vi "zad2a.vi"() -> ()   [LabVIEW 2017]
uses:
  zad2Zmienna.vi
panel:
  out "Numeric":dbl
  in  "OK Button":bool
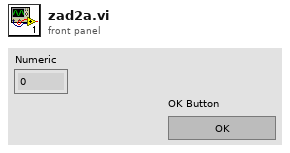
[diagram p1: front panel]
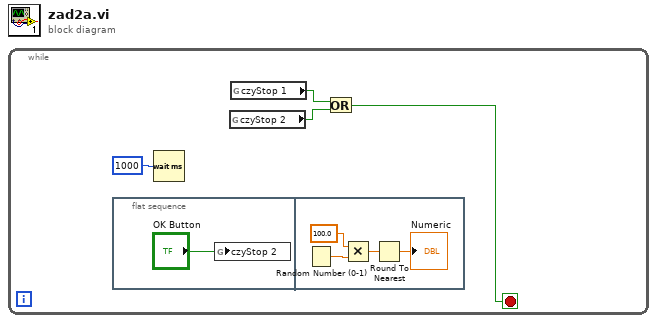
[diagram p0: block diagram]
diagram:
  n1 = while {
    stop <- w1 stop-if-true
    n2 = flat-sequence {
      frame #0 {
        n3 = global write "zad2Zmienna.vi" "czyStop 2"("OK Button") -> ()
      }
      frame #1 {
        n4 = Random Number (0-1)() -> (number: 0 to 1=w7:dbl)
        n5 = Multiply(x=100.0, y=w7) -> (x*y=w8:dbl)
        n6 = Round To Nearest(number=w8) -> (nearest integer value=→"Numeric":dbl)
      }
    }
    n7 = Wait (ms)(milliseconds to wait=u32 1000) -> ()  [unwired: 1 out]
    n8 = global read "zad2Zmienna.vi" "czyStop 2"() -> (w3:bool)
    n9 = global read "zad2Zmienna.vi" "czyStop 1"() -> (w2:bool)
    n10 = Or(x=w2, y=w3) -> (x .or. y?=w1:bool)
  }
